vi "decodeStream.vi"(8 "error in (no error)":errorcluster, 9 "beginIndex":i32, 10 "binary stream":u8[](array[numeric]), 11 "tBSONJavaScriptWithScope in":refnum<class "tBSONJavaScriptWithScope.lvclass">) -> (0 "error out":errorcluster, 1 "endIndex":i32, 2 "binary stream out":u8[](array[numeric]), 3 "tBSONJavaScriptWithScope out":refnum<class "tBSONJavaScriptWithScope.lvclass">)   [LabVIEW 2013, in "BSON.lvlib" / "tBSONJavaScriptWithScope.lvclass"]
uses:
  tBSONJavaScriptWithScope.lvclass
  status.ctl
  tBSONElement/setName.vi
  tBSONJavaScript/setScript.vi
  setScope.vi
  BSON.lvlib
  tBSONDocument/tBSONDocument.lvclass
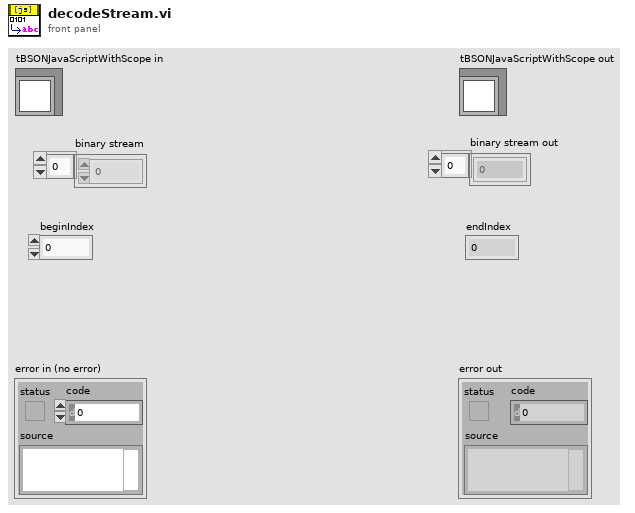
[diagram p1: front panel]
types:
  T1 = typedef "BSON.lvlib/status.ctl" = enum16{"Stream Corrupted or Ended Abruptly", "Incorrect Type In Stream", "ObjectID Invalid", "Method Not Implemented", "Invalid Name", "Invalid URI", "AutoReconnect", "Operation Failed", "Incorrectly Configured", "Cursor Not Found", "Timeout", "Invalid Type", "Empty Name", "Duplicate Name", "MD5Incorrect"}
  T2 = typedef "BSON.lvlib/tBSONElement.lvclass/type.ctl" = u8
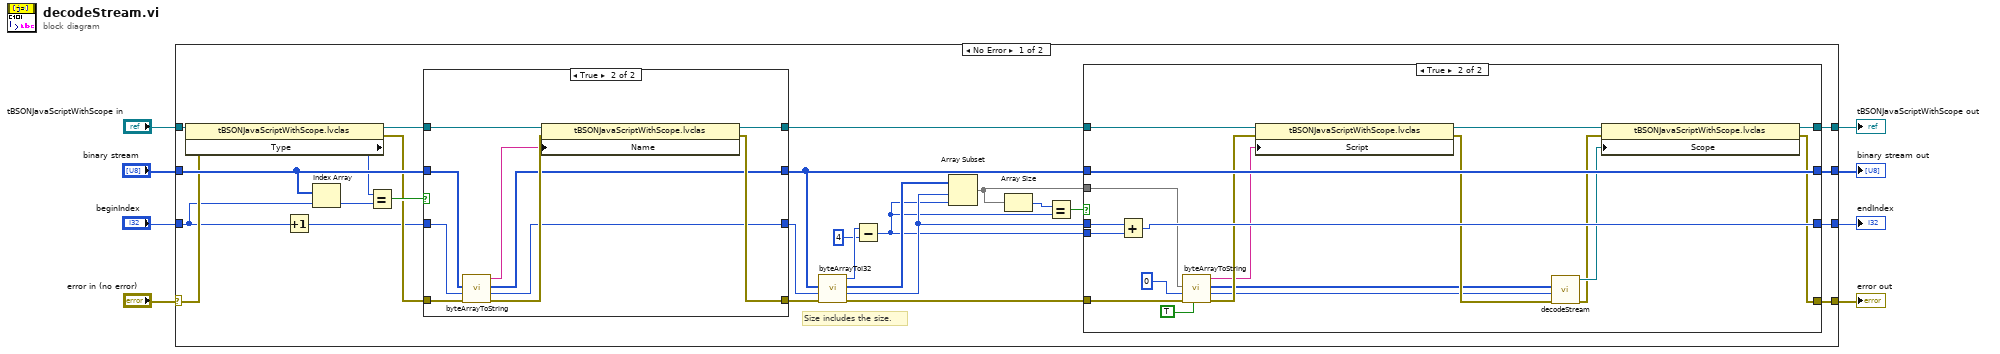
[diagram p0: block diagram]
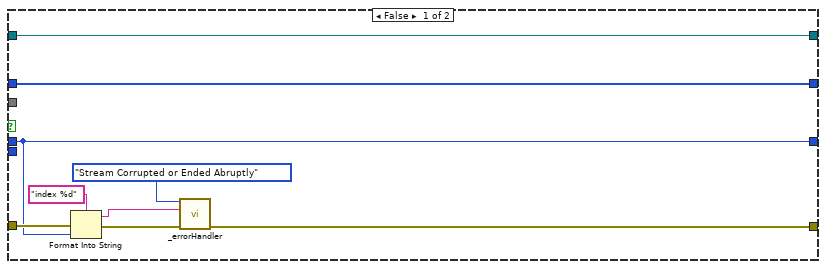
[diagram p2: hidden frame]
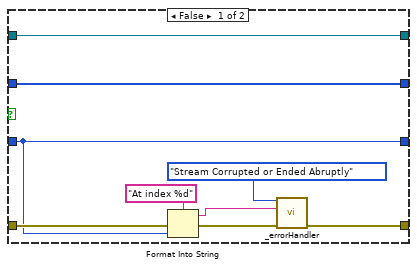
[diagram p3: hidden frame]
diagram:
  n1 = case shown="No Error" "error in (no error)" {
    selector: "error in (no error)" -> [w31 w86]
    tunnel: [w18 w86] -> w3
    tunnel: [w19 w85] -> w2
    tunnel: "tBSONJavaScriptWithScope in" -> [w33 w85]
    tunnel: "binary stream" -> [w35 w83]
    tunnel: "beginIndex" -> [w10 w84]
    tunnel: [w16 w84] -> w4
    tunnel: [w20 w83] -> w1
    frame No Error {
      # "Size includes the size."
      n2 = property class="tBSONJavaScriptWithScope.lvclas"(reference=w33, error in=w31) -> (reference out=w32:refnum<class "tBSONJavaScriptWithScope.lvclass">, error out=w28:errorcluster, "Type"=w30:T2)
      n3 = Increment(x=w10) -> (x+1=w9:i32)
      n4 = Index Array(array=w35, index=w10) -> (element=w34:u8)
      n5 = Equal?(x=w30, y=w34) -> (x = y?=w29:bool)
      n6 = case shown="True" w29 {
        tunnel: [w71 w82] -> w27
        tunnel: [w65 w77] -> w26
        tunnel: [w70 w81] -> w23
        tunnel: w35 -> [w64 w74]
        tunnel: w32 -> [w70 w80]
        tunnel: w9 -> [w65 w76]
        tunnel: w28 -> [w69 w79]
        tunnel: [w64 w73] -> w21
        frame False {
          n7 = Format Into String(format string="At index %d", error in=w69, w65) -> (resulting string=w66:string, error out=w67:errorcluster)  [unwired: 1 in]
          n8 = call "_errorHandler.vi"("error in (no error)"=w67, "Additional Text"=w66, "Error Type"=status."Stream Corrupted or Ended Abruptly") -> ("error out"=w71:errorcluster)  [unwired: 8 in]
        }
        frame True {
          n9 = call "byteArrayToString.vi"("error in (no error)"=w79, "startIndex"=w76, "ByteArrayIn"=w74) -> ("error out"=w78:errorcluster, "endIndex"=w77:i32, "ByteArrayOut"=w73:u8[], "String"=w75:string)  [unwired: 5 in]
          n10 = property class="tBSONJavaScriptWithScope.lvclas"(reference=w80, error in=w78, "Name"=w75) -> (reference out=w81:refnum<class "tBSONJavaScriptWithScope.lvclass">, error out=w82:errorcluster)
        }
      }
      n11 = call "byteArrayToI32.vi"("error in (no error)"=w27, "StartIndex"=w26, "ByteArrayIn"=w21) -> ("error out"=w15:errorcluster, "EndIndex"=w17:i32, "ByteArrayOut"=w25:u8[], "I32"=w13:i32)  [unwired: 5 in]
      n12 = Subtract(x=w13, y=4) -> (x-y=w11:i32)
      n13 = Array Subset(array=w25, index=w17, length=w11) -> (w14:u8[])
      n14 = Array Size(array=w14) -> (size(s)=w24:i32)
      n15 = Equal?(x=w24, y=w11) -> (x = y?=w22:bool)
      n16 = case shown="True" w22 {
        tunnel: w23 -> [w39 w55]
        tunnel: w21 -> [w40 w63]
        tunnel: [w40 w63] -> w20
        tunnel: [w39 w49] -> w19
        tunnel: [w38 w45] -> w18
        tunnel: w17 -> [w36 w62]
        tunnel: [w36 w60] -> w16
        tunnel: w15 -> [w37 w59]
        tunnel: w14 -> [_ w58]
        tunnel: w11 -> [_ w61]
        frame False {
          n17 = Format Into String(format string="index %d", error in=w37, w36) -> (resulting string=w44:string, error out=w43:errorcluster)  [unwired: 1 in]
          n18 = call "_errorHandler.vi"("error in (no error)"=w43, "Additional Text"=w44, "Error Type"=status."Stream Corrupted or Ended Abruptly") -> ("error out"=w38:errorcluster)  [unwired: 8 in]
        }
        frame True {
          n19 = Add(x=w62, y=w61) -> (x+y=w60:i32)
          n20 = call "byteArrayToString.vi"("lengthPrepended"=TRUE, "error in (no error)"=w59, "startIndex"=0, "ByteArrayIn"=w58) -> ("error out"=w54:errorcluster, "endIndex"=w50:i32, "ByteArrayOut"=w51:u8[], "String"=w53:string)  [unwired: 4 in]
          n21 = property class="tBSONJavaScriptWithScope.lvclas"(reference=w55, error in=w54, "Script"=w53) -> (reference out=w48:refnum<class "tBSONJavaScriptWithScope.lvclass">, error out=w52:errorcluster)
          n22 = call "decodeStream.vi"("error in (no error)"=w52, "Begin Index"=w50, "Byte Data In"=w51) -> ("error out"=w46:errorcluster, "tBSONDocument out"=w47:refnum<class "tBSONDocument.lvclass">)  [unwired: 5 in, 2 out]
          n23 = property class="tBSONJavaScriptWithScope.lvclas"(reference=w48, error in=w46, "Scope"=w47) -> (reference out=w49:refnum<class "tBSONJavaScriptWithScope.lvclass">, error out=w45:errorcluster)
        }
      }
    }
    frame Error {
    }
  }
  "error out" <- w3
  "tBSONJavaScriptWithScope out" <- w2
  "binary stream out" <- w1
  "endIndex" <- w4
